vi "Make Channels Coincident Low.vi"(8 "interp. method":i32(ring) items=["nearest", "linear", "spline", "cubic Hermite", "Lagrange"], 9 "Cluster 2":T1={"Colour"=0, "Inst type"=enum."Pitot-static tube", "Inst name"="Manometer voltage", "Symbol"="U", "Code name"="", "Extra Info"="U", "Inst Array"=enum."PWA", "Index"=0, "Voltage Index"=0, "Extra Titles"=[], "Extra Values"=[], "Eng Values"=[], "Time (ms)"=[], "TT / Voltage"=[], "U"=0.0, "u^2"=0.0, "u^3"=0.0, "u^4"=0.0, "Skew_u"=0.0, "Kurt_u"=0.0, "Sd Error in Mean"=0.0, "% u'/U"=0.0, "X"=0.0, "Y"=0.0, "Z"=0.0, "Spectra"={"First Name"="", "Second Name"="", "X axis name"="", "Y axis name"="", "X array"=[], "Y array"=[]}, "Autocorrelation"={"First Name"="", "Second Name"="", "X axis name"="", "Y axis name"="", "X array"=[], "Y array"=[]}, "Timescale integral to 25%"=0.0, "Sd Error in Variance"=0.0, "Calib File"=path "", "Calib Constants"=[], "Histogram"={"First Name"="", "Second Name"="", "X axis name"="", "Y axis name"="", "X array"=[], "Y array"=[]}, "Output Position"=FALSE, "Full Stats"=FALSE} {"Sd Error in Variance" format="%.2f"; "Skew_u" format="%.2f"; "% u'/U" format="%.2f"; "Sd Error in Mean" format="%.2f"; "Kurt_u" format="%.2f"; "u^4" format="%.2f"; "u^3" format="%.2f"; "U" format="%.2f"; "u^2" format="%.2f"}, 11 "Cluster 1":T1={"Colour"=0, "Inst type"=enum."Pitot-static tube", "Inst name"="Manometer voltage", "Symbol"="U", "Code name"="", "Extra Info"="U", "Inst Array"=enum."PWA", "Index"=0, "Voltage Index"=0, "Extra Titles"=[], "Extra Values"=[], "Eng Values"=[], "Time (ms)"=[], "TT / Voltage"=[], "U"=0.0, "u^2"=0.0, "u^3"=0.0, "u^4"=0.0, "Skew_u"=0.0, "Kurt_u"=0.0, "Sd Error in Mean"=0.0, "% u'/U"=0.0, "X"=0.0, "Y"=0.0, "Z"=0.0, "Spectra"={"First Name"="", "Second Name"="", "X axis name"="", "Y axis name"="", "X array"=[], "Y array"=[]}, "Autocorrelation"={"First Name"="", "Second Name"="", "X axis name"="", "Y axis name"="", "X array"=[], "Y array"=[]}, "Timescale integral to 25%"=0.0, "Sd Error in Variance"=0.0, "Calib File"=path "", "Calib Constants"=[], "Histogram"={"First Name"="", "Second Name"="", "X axis name"="", "Y axis name"="", "X array"=[], "Y array"=[]}, "Output Position"=FALSE, "Full Stats"=FALSE} {"Sd Error in Variance" format="%.2f"; "Skew_u" format="%.2f"; "% u'/U" format="%.2f"; "Sd Error in Mean" format="%.2f"; "Kurt_u" format="%.2f"; "u^4" format="%.2f"; "u^3" format="%.2f"; "U" format="%.2f"; "u^2" format="%.2f"}) -> (1 "Coincident Channel 2":T1={"Colour"=0, "Inst type"=enum."Pitot-static tube", "Inst name"="Manometer voltage", "Symbol"="U", "Code name"="", "Extra Info"="U", "Inst Array"=enum."PWA", "Index"=0, "Voltage Index"=0, "Extra Titles"=[], "Extra Values"=[], "Eng Values"=[], "Time (ms)"=[], "TT / Voltage"=[], "U"=0.0, "u^2"=0.0, "u^3"=0.0, "u^4"=0.0, "Skew_u"=0.0, "Kurt_u"=0.0, "Sd Error in Mean"=0.0, "% u'/U"=0.0, "X"=0.0, "Y"=0.0, "Z"=0.0, "Spectra"={"First Name"="", "Second Name"="", "X axis name"="", "Y axis name"="", "X array"=[], "Y array"=[]}, "Autocorrelation"={"First Name"="", "Second Name"="", "X axis name"="", "Y axis name"="", "X array"=[], "Y array"=[]}, "Timescale integral to 25%"=0.0, "Sd Error in Variance"=0.0, "Calib File"=path "", "Calib Constants"=[], "Histogram"={"First Name"="", "Second Name"="", "X axis name"="", "Y axis name"="", "X array"=[], "Y array"=[]}, "Output Position"=FALSE, "Full Stats"=FALSE} {"Sd Error in Variance" format="%.2f"; "Skew_u" format="%.2f"; "% u'/U" format="%.2f"; "Sd Error in Mean" format="%.2f"; "Kurt_u" format="%.2f"; "u^4" format="%.2f"; "u^3" format="%.2f"; "U" format="%.2f"; "u^2" format="%.2f"}, 3 "Coincident Channel 1":T1={"Colour"=0, "Inst type"=enum."Pitot-static tube", "Inst name"="Manometer voltage", "Symbol"="U", "Code name"="", "Extra Info"="U", "Inst Array"=enum."PWA", "Index"=0, "Voltage Index"=0, "Extra Titles"=[], "Extra Values"=[], "Eng Values"=[], "Time (ms)"=[], "TT / Voltage"=[], "U"=0.0, "u^2"=0.0, "u^3"=0.0, "u^4"=0.0, "Skew_u"=0.0, "Kurt_u"=0.0, "Sd Error in Mean"=0.0, "% u'/U"=0.0, "X"=0.0, "Y"=0.0, "Z"=0.0, "Spectra"={"First Name"="", "Second Name"="", "X axis name"="", "Y axis name"="", "X array"=[], "Y array"=[]}, "Autocorrelation"={"First Name"="", "Second Name"="", "X axis name"="", "Y axis name"="", "X array"=[], "Y array"=[]}, "Timescale integral to 25%"=0.0, "Sd Error in Variance"=0.0, "Calib File"=path "", "Calib Constants"=[], "Histogram"={"First Name"="", "Second Name"="", "X axis name"="", "Y axis name"="", "X array"=[], "Y array"=[]}, "Output Position"=FALSE, "Full Stats"=FALSE} {"Sd Error in Variance" format="%.2f"; "Skew_u" format="%.2f"; "% u'/U" format="%.2f"; "Sd Error in Mean" format="%.2f"; "Kurt_u" format="%.2f"; "u^4" format="%.2f"; "u^3" format="%.2f"; "U" format="%.2f"; "u^2" format="%.2f"})   [LabVIEW 2011]
uses:
  Controls/Analysis_info_cluster.ctl
  Controls/Inst_type.ctl
  Controls/Instrument_Array.ctl
  Controls/XY_Plot_Cluster.ctl
  <vilib>/gmath/NI_Gmath.lvlib
  Globals/LDA_meas_global_1.vi
panel:
  out "Ref size":i32
  out "Interp size":i32
  out "U1 and U2 Raw":cluster{"yi":dbl[], "yi":dbl[]}[](graph)
  out "U1 and U2 made coincident":cluster{"yi":dbl[], "yi":dbl[]}[](graph)
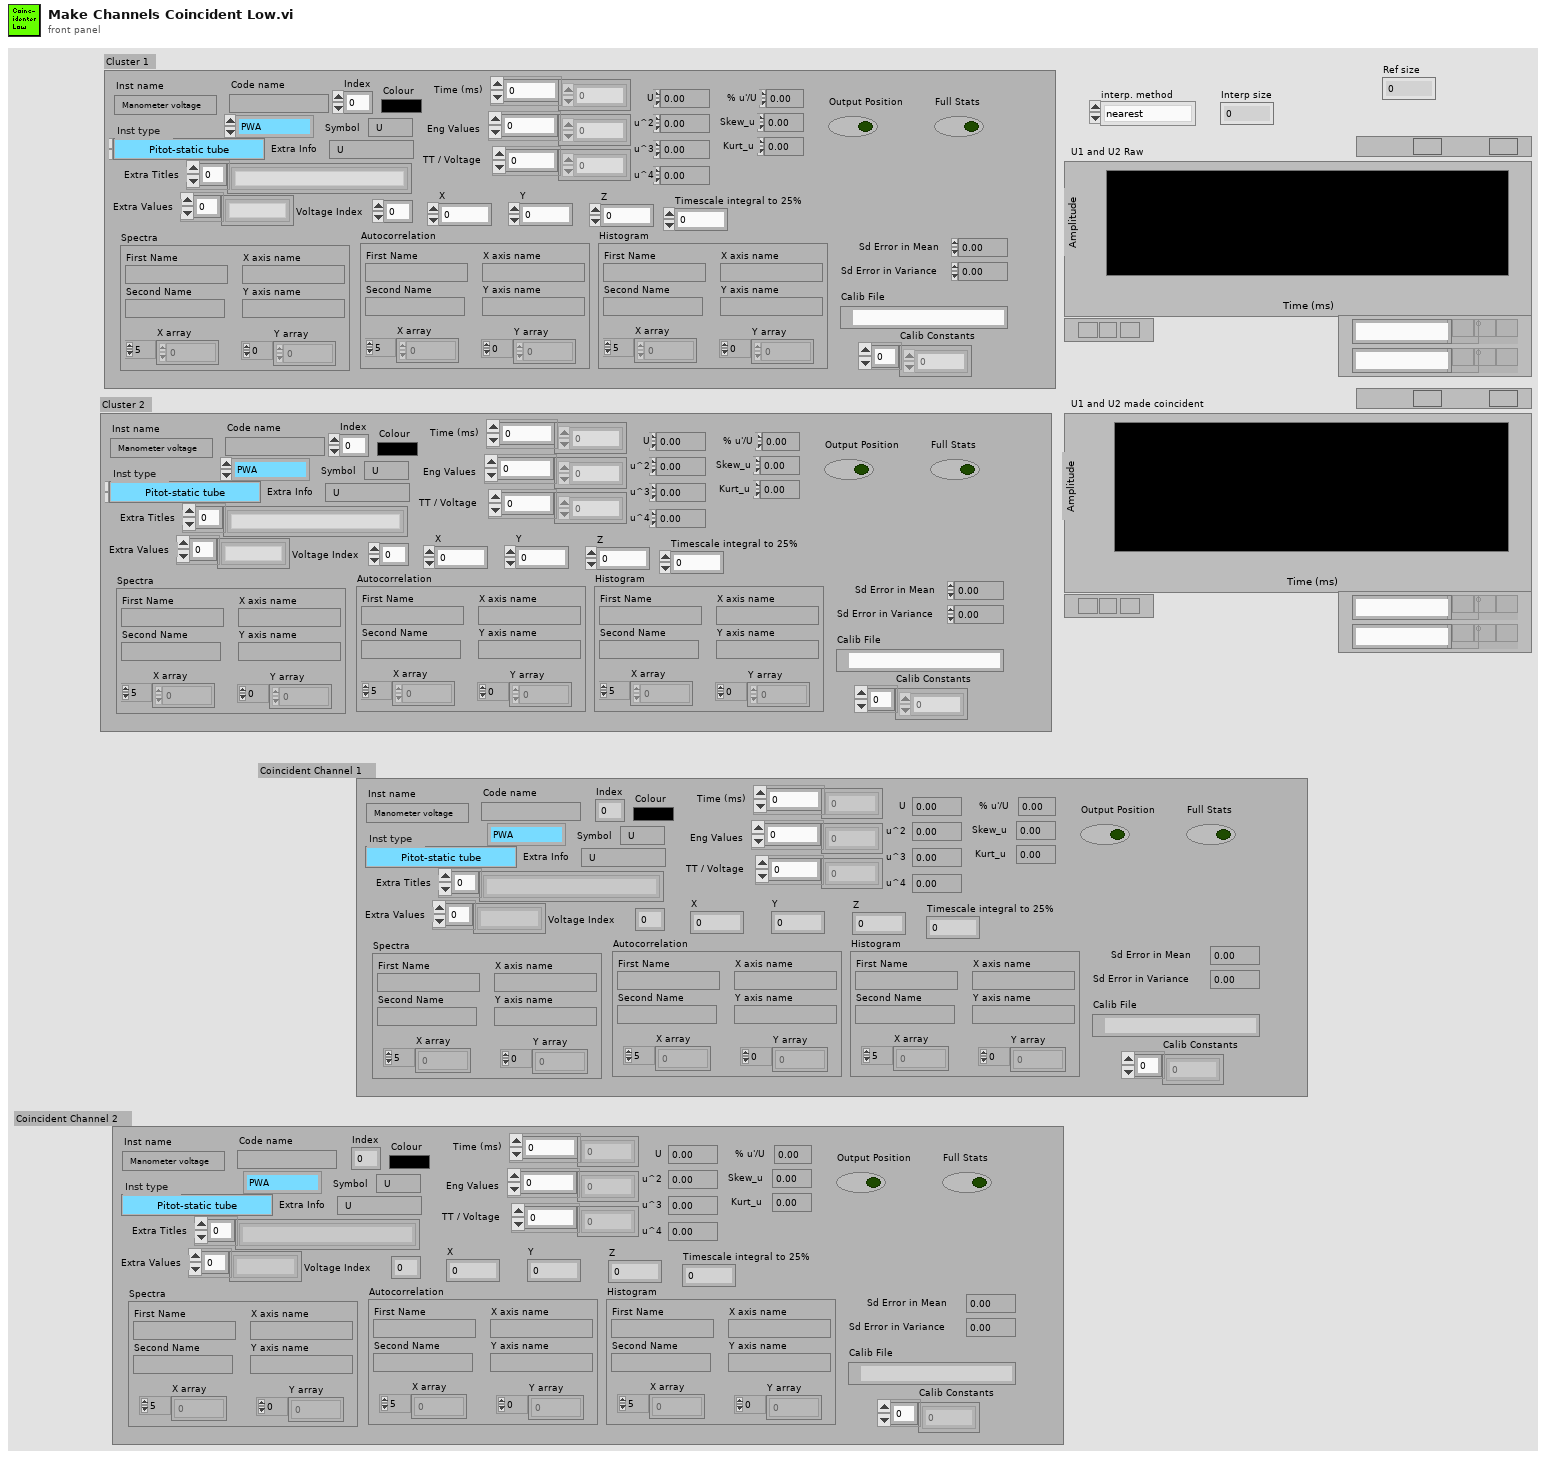
[diagram p1: front panel]
types:
  T1 = typedef "Analysis_info_cluster.ctl" = cluster{"Colour":u32, "Inst type":T2, "Inst name":string, "Symbol":string, "Code name":string, "Extra Info":string, "Inst Array":T3, "Index":i32, "Voltage Index":i32, "Extra Titles":string[], "Extra Values":string[], "Eng Values":dbl[], "Time (ms)":dbl[], "TT / Voltage":dbl[], "U":dbl, "u^2":dbl, "u^3":dbl, "u^4":dbl, "Skew_u":dbl, "Kurt_u":dbl, "Sd Error in Mean":dbl, "% u'/U":dbl, "X":dbl, "Y":dbl, "Z":dbl, "Spectra":T4, "Autocorrelation":T4, "Timescale integral to 25%":dbl, "Sd Error in Variance":dbl, "Calib File":path, "Calib Constants":dbl[], "Histogram":T4, "Output Position":bool, "Full Stats":bool}
  T2 = typedef "Inst_type.ctl" = enum16{"Propeller anemometer", "Raw voltage", "Pressure Transducer", "Pitot-static tube", "Preston tube", "Hot wire", "Cross wire 1", "Cross wire 2", "Generic Linear", "Generic Polynomial", "Generic BackPoly", "Fast FID", "Thermocouple", "Cold wire", "Pulsed Wire", "LDA Vel", "LDA Tran time", "LDA Arr time"}
  T3 = typedef "Instrument_Array.ctl" = enum16{"PWA", "LDA", "Analogue"}
  T4 = typedef "XY_Plot_Cluster.ctl" = cluster{"First Name":string, "Second Name":string, "X axis name":string, "Y axis name":string, "X array":dbl[], "Y array":dbl[]}
  T5 = cluster{"Time (ms)":dbl[], "Eng Values":dbl[], "TT / Voltage":dbl[]}
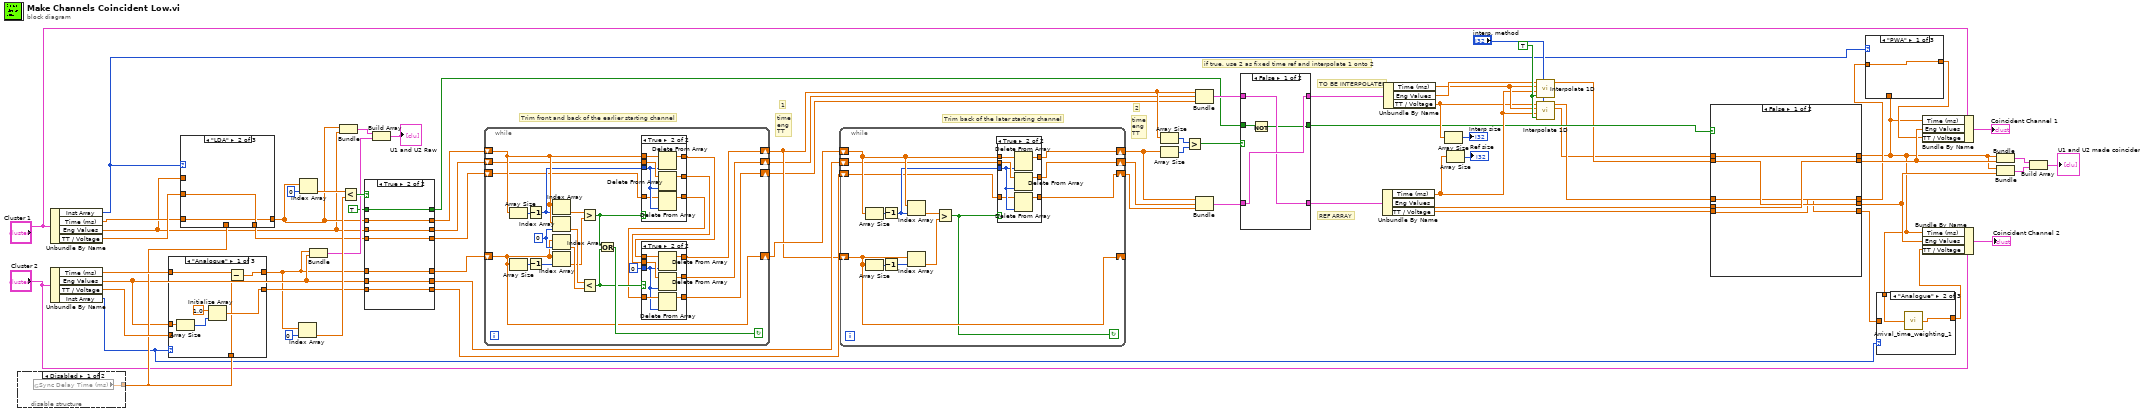
[diagram p0: block diagram]
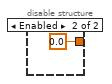
[diagram p2: hidden frame]
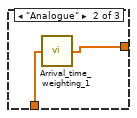
[diagram p3: hidden frame]
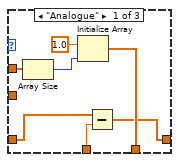
[diagram p9: hidden frame]
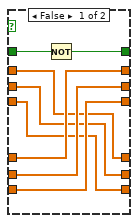
[diagram p14: hidden frame]
diagram:
  w46 = TRUE ("X is monotonic")
  # "Trim back of the later starting channel"
  # "Trim front and back of the earlier starting channel"
  # "TO BE INTERPOLATED"
  # "REF ARRAY"
  # "if true, use 2 as fixed time ref and interpolate 1 onto 2"
  # "2"
  # "1"
  # "time\neng\nTT"
  # "time\neng\nTT"
  n1 = disable-structure shown="Disabled" {
    disable-tunnel: [w72 0.0 ("Sync Delay Time (ms)")] -> w13
    frame Disabled {
      n2 = global read "LDA_meas_global_1.vi" "Sync Delay Time (ms)"() -> (w72:dbl)
    }
    frame Enabled {
    }
  }
  n3 = Unbundle By Name("Cluster 1") -> ("Inst Array"=w4:T3, "Time (ms)"=w14:dbl[], "Eng Values"=w11:dbl[], "TT / Voltage"=w25:dbl[])
  n4 = Unbundle By Name("Cluster 2") -> ("Time (ms)"=w15:dbl[], "Eng Values"=w10:dbl[], "TT / Voltage"=w17:dbl[], "Inst Array"=w7:T3)
  n5 = case shown="\"Analogue\"" w7 {
    tunnel: w17 -> [_ w82 w84]
    tunnel: [w77 w82 w84] -> w16
    tunnel: w10 -> [w78 _ _]
    tunnel: w13 -> [w76 _ _]
    tunnel: w15 -> [w75 w81 w83]
    tunnel: [w74 w81 w83] -> w9
    frame "Analogue" {
      n6 = Array Size(array=w78) -> (size(s)=w79:i32)
      n7 = Initialize Array(1.0 ("element"), w79) -> (w77:dbl[])
      n8 = Subtract(x=w75, y=w76) -> (x-y=w74:dbl[])
    }
    frame "LDA" {
    }
    frame "PWA" {
    }
  }
  n9 = case shown="\"LDA\"" w4 {
    tunnel: [w88 w93 w95] -> w26
    tunnel: w25 -> [_ w93 w95]
    tunnel: w11 -> [w90 _ _]
    tunnel: [w86 w92 w94] -> w12
    tunnel: w14 -> [w87 w92 w94]
    tunnel: w13 -> [w85 _ _]
    frame "Analogue" {
      n10 = Array Size(array=w90) -> (size(s)=w89:i32)
      n11 = Initialize Array(1.0 ("element"), w89) -> (w88:dbl[])
      n12 = Subtract(x=w87, y=w85) -> (x-y=w86:dbl[])
    }
    frame "LDA" {
    }
    frame "PWA" {
    }
  }
  n13 = Index Array(array=w9, index=0) -> (element=w68:dbl)
  n14 = Index Array(array=w12, index=0) -> (element=w69:dbl)
  n15 = Bundle("Time (ms)"=w9, "Eng Values"=w10) -> (w39:cluster{"Time (ms)":dbl[], "Eng Values":dbl[]})  [unwired: 1 in]
  n16 = Bundle("Time (ms)"=w12, "Eng Values"=w11) -> (w33:cluster{"Time (ms)":dbl[], "Eng Values":dbl[]})  [unwired: 1 in]
  n17 = Less?(x=w69, y=w68) -> (x < y?=w67:bool)
  n18 = case shown="True" w67 {
    tunnel: w12 -> [w98 w110]
    tunnel: [w103 w110] -> w66
    tunnel: [w102 w109] -> w65
    tunnel: w11 -> [w99 w109]
    tunnel: [w101 w108] -> w64
    tunnel: w26 -> [w100 w108]
    tunnel: [w98 w107] -> w63
    tunnel: w9 -> [w103 w107]
    tunnel: [w99 w106] -> w61
    tunnel: w10 -> [w102 w106]
    tunnel: [w100 w105] -> w60
    tunnel: w16 -> [w101 w105]
    tunnel: TRUE -> [w97 w104]
    tunnel: [w96 w104] -> w28
    frame False {
      n19 = Not(x=w97) -> (.not. x?=w96:bool)
    }
    frame True {
    }
  }
  n20 = Build Array(w33, w39) -> (→"U1 and U2 Raw":cluster{"Time (ms)":dbl[], "Eng Values":dbl[]}[])
  n21 = while {
    shift-right: [w121] -> w54
    shift-left: w66 -> [w126]
    shift-right: [w120] -> w53
    shift-left: w65 -> [w125]
    shift-right: [w111] -> w62
    shift-left: w63 -> [w111]
    shift-right: [w112] -> w52
    shift-left: w64 -> [w114]
    stop <- w127 continue-if-true
    w133 = 0 ("index")
    n22 = Array Size(array=w126) -> (size(s)=w118:i32)
    n23 = Array Size(array=w111) -> (size(s)=w116:i32)
    n24 = Decrement(x=w118) -> (x-1=w117:i32)
    n25 = Decrement(x=w116) -> (x-1=w115:i32)
    n26 = Index Array(array=w126, index=w117) -> (element=w130:dbl)
    n27 = Index Array(array=w126, index=w133) -> (element=w132:dbl)
    n28 = Index Array(array=w111, index=w133) -> (element=w131:dbl)
    n29 = Index Array(array=w111, index=w115) -> (element=w129:dbl)
    n30 = Greater?(x=w130, y=w129) -> (0:w128:bool)
    n31 = Less?(x=w132, y=w131) -> (x < y?=w124:bool)
    n32 = Or(x=w128, y=w124) -> (x .or. y?=w127:bool)
    n33 = case shown="True" w128 {
      tunnel: w126 -> [w146 w152]
      tunnel: w125 -> [w145 w153]
      tunnel: w117 -> [_ w149]
      tunnel: [w146 w151] -> w123
      tunnel: [w145 w150] -> w122
      tunnel: [w144 w148] -> w113
      tunnel: w114 -> [w144 w147]
      frame False {
      }
      frame True {
        n34 = Delete From Array(array=w152, index=w149) -> (array with subset deleted=w151:dbl[])  [unwired: 1 in, 1 out]
        n35 = Delete From Array(array=w153, index=w149) -> (array with subset deleted=w150:dbl[])  [unwired: 1 in, 1 out]
        n36 = Delete From Array(array=w147, index=w149) -> (array with subset deleted=w148:dbl[])  [unwired: 1 in, 1 out]
      }
    }
    n37 = case shown="True" w124 {
      tunnel: w123 -> [w136 w142]
      tunnel: w122 -> [w135 w143]
      tunnel: 0 -> [_ w137]
      tunnel: [w136 w141] -> w121
      tunnel: [w135 w140] -> w120
      tunnel: w113 -> [w134 w139]
      tunnel: [w134 w138] -> w112
      frame False {
      }
      frame True {
        n38 = Delete From Array(array=w142, index=w137) -> (array with subset deleted=w141:dbl[])  [unwired: 1 in, 1 out]
        n39 = Delete From Array(array=w143, index=w137) -> (array with subset deleted=w140:dbl[])  [unwired: 1 in, 1 out]
        n40 = Delete From Array(array=w139, index=w137) -> (array with subset deleted=w138:dbl[])  [unwired: 1 in, 1 out]
      }
    }
  }
  n41 = while {
    shift-right: [w156] -> w55
    shift-left: w62 -> [w165]
    shift-right: [w155] -> w56
    shift-left: w61 -> [w164]
    shift-right: [w158] -> _
    shift-left: w54 -> [w158]
    shift-right: [w154] -> w57
    shift-left: w60 -> [w159]
    stop <- w157 continue-if-true
    n42 = Array Size(array=w165) -> (size(s)=w163:i32)
    n43 = Array Size(array=w158) -> (size(s)=w161:i32)
    n44 = Decrement(x=w163) -> (x-1=w162:i32)
    n45 = Decrement(x=w161) -> (x-1=w160:i32)
    n46 = Index Array(array=w165, index=w162) -> (element=w167:dbl)
    n47 = Index Array(array=w158, index=w160) -> (element=w166:dbl)
    n48 = Greater?(x=w167, y=w166) -> (0:w157:bool)
    n49 = case shown="True" w157 {
      tunnel: w165 -> [w170 w176]
      tunnel: w164 -> [w169 w177]
      tunnel: w162 -> [_ w173]
      tunnel: [w170 w175] -> w156
      tunnel: [w169 w174] -> w155
      tunnel: [w168 w172] -> w154
      tunnel: w159 -> [w168 w171]
      frame False {
      }
      frame True {
        n50 = Delete From Array(array=w176, index=w173) -> (array with subset deleted=w175:dbl[])  [unwired: 1 in, 1 out]
        n51 = Delete From Array(array=w177, index=w173) -> (array with subset deleted=w174:dbl[])  [unwired: 1 in, 1 out]
        n52 = Delete From Array(array=w171, index=w173) -> (array with subset deleted=w172:dbl[])  [unwired: 1 in, 1 out]
      }
    }
  }
  n53 = Array Size(array=w54) -> (size(s)=w59:i32)
  n54 = Array Size(array=w55) -> (size(s)=w58:i32)
  n55 = Greater?(x=w59, y=w58) -> (0:w34:bool)
  n56 = Bundle("Time (ms)"=w54, "Eng Values"=w53, "TT / Voltage"=w52) -> (w51:T5)  [unwired: 1 in]
  n57 = Bundle("Time (ms)"=w55, "Eng Values"=w56, "TT / Voltage"=w57) -> (w50:T5)  [unwired: 1 in]
  n58 = case shown="False" w34 {
    tunnel: w51 -> [w180 w183]
    tunnel: w50 -> [w181 w184]
    tunnel: [w180 w184] -> w48
    tunnel: [w181 w183] -> w49
    tunnel: [w178 w182] -> w29
    tunnel: w28 -> [w179 w182]
    frame False {
      n59 = Not(x=w179) -> (.not. x?=w178:bool)
    }
    frame True {
    }
  }
  n60 = Unbundle By Name(w48) -> ("Time (ms)"=w38:dbl[], "Eng Values"=w22:dbl[], "TT / Voltage"=w21:dbl[])
  n61 = Unbundle By Name(w49) -> ("Time (ms)"=w41:dbl[], "Eng Values"=w45:dbl[], "TT / Voltage"=w37:dbl[])
  n62 = Array Size(array=w37) -> (size(s)=→"Interp size":i32)
  n63 = Array Size(array=w38) -> (size(s)=→"Ref size":i32)
  n64 = call <vilib>:"Interpolate 1D.vi"("method"="interp. method", "X is monotonic"=w46, "xi"=w38, "X"=w41, "Y"=w45) -> ("yi"=w24:dbl[])  [unwired: 1 in, 5 out]
  n65 = call <vilib>:"Interpolate 1D.vi"("method"="interp. method", "X is monotonic"=w46, "xi"=w38, "X"=w41, "Y"=w37) -> ("xi used"=w20:dbl[], "yi"=w23:dbl[])  [unwired: 1 in, 4 out]
  n66 = case shown="False" w29 {
    tunnel: [w189 w194] -> w1
    tunnel: w20 -> [w189 w194]
    tunnel: [w188 w193] -> w19
    tunnel: w24 -> [w187 w193]
    tunnel: w23 -> [w185 w192]
    tunnel: [w186 w192] -> w3
    tunnel: w22 -> [w188 w191]
    tunnel: [w187 w191] -> w18
    tunnel: [w185 w190] -> w5
    tunnel: w21 -> [w186 w190]
    tunnel: w20 -> [_ _]
    frame False {
    }
    frame True {
    }
  }
  n67 = case shown="\"PWA\"" w4 {
    tunnel: [w195 w197 w198] -> w2
    tunnel: w3 -> [w195 _ w198]
    tunnel: w1 -> [_ w196 _]
    frame "PWA" {
    }
    frame "Analogue" {
      n68 = call "Arrival_time_weighting_1.vi"("Arrival times"=w196) -> ("Weighting"=w197:dbl[])
    }
    frame "LDA" {
    }
  }
  n69 = case shown="\"Analogue\"" w7 {
    tunnel: [w199 w201 w202] -> w6
    tunnel: w5 -> [w199 _ w202]
    tunnel: w1 -> [_ w200 _]
    frame "PWA" {
    }
    frame "Analogue" {
      n70 = call "Arrival_time_weighting_1.vi"("Arrival times"=w200) -> ("Weighting"=w201:dbl[])
    }
    frame "LDA" {
    }
  }
  n71 = Bundle By Name(cluster="Cluster 1", "Time (ms)"=w1, "Eng Values"=w19, "TT / Voltage"=w2) -> (→"Coincident Channel 1":T1)
  n72 = Bundle By Name(cluster="Cluster 2", "Time (ms)"=w1, "Eng Values"=w18, "TT / Voltage"=w6) -> (→"Coincident Channel 2":T1)
  n73 = Bundle("xi used"=w1, "yi"=w19) -> (w43:cluster{"xi used":dbl[], "yi":dbl[]})  [unwired: 1 in]
  n74 = Bundle("xi used"=w1, "Eng Values"=w18) -> (w44:cluster{"xi used":dbl[], "Eng Values":dbl[]})  [unwired: 1 in]
  n75 = Build Array(w43, w44) -> (→"U1 and U2 made coincident":cluster{"xi used":dbl[], "Eng Values":dbl[]}[])
